vi "PhotonCamera_GetFPSLimit.vi"(9 "BaseNTName":string="/photonvision", 11 "CameraName":string) -> (0 "error out":errorcluster, 3 "FPSLimit":i32)   [LabVIEW 2019, in "PhotonVisionLib.lvlib"]
doc: "Gets the FPS (Frame Per Second) limit set on the camera.\n\nInputs:\n - CameraName -- The nickname of the camera (found in the PhotonVision UI).\n - BaseNTName - string - Base Nework Table name. (Optional. Default: /photonvision )\n \nOutputs:\n - FPSLimit -- integer -- The current FPS limit. ( -1 indicates unlimited )\n - Error Out -- Contains error information if a Network table ot other error occured."
uses:
  PhotonVisionLib.lvlib
  <vilib>/Rock Robotics/Network Tables/NT Read Integer.vi
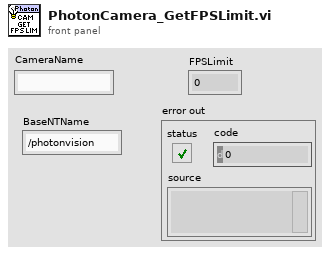
[diagram p1: front panel]
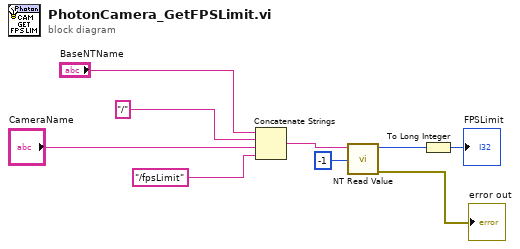
[diagram p0: block diagram]
diagram:
  n1 = Concatenate Strings("BaseNTName", "/", "CameraName", "/fpsLimit") -> (w6:string)
  n2 = call-poly <vilib>:"NT Read Value.vi"("default value"=i64 -1 ("Default Value"), "name"=w6) -> ("error out"=→"error out":errorcluster, "value"=w1:i64)  [unwired: 7 in, 1 out]
  n3 = To Long Integer(number=w1) -> (32bit integer=→"FPSLimit":i32)
